vi "Error - Process.vi"(8 "error in (no error)":errorcluster, 11 "View Model":T1) -> (0 "error out":errorcluster)   [LabVIEW 2017]
doc: "Template for creating process"
uses:
  View Model/Controls/View Model.ctl
  Controls/Error Model.ctl
  Controls/Error EventData.ctl
  Controls/Error Type.ctl
  Elevator Controller/Controls/Elevator Model.ctl
  Elevator Controller/Controls/Elevator Overhead.ctl
  Elevator Controller/Controls/Elevator States.ctl
  Elevator Controller/Controls/Elevator Location.ctl
  Elevator Controller/Controls/Elevator Command Event.ctl
  Elevator Controller/Controls/Elevator Commands.ctl
  Configuration/Controls/Configuration Model.ctl
  Configuration/Controls/Configuration Data.ctl
  View Model/Controls/Shared Model.ctl
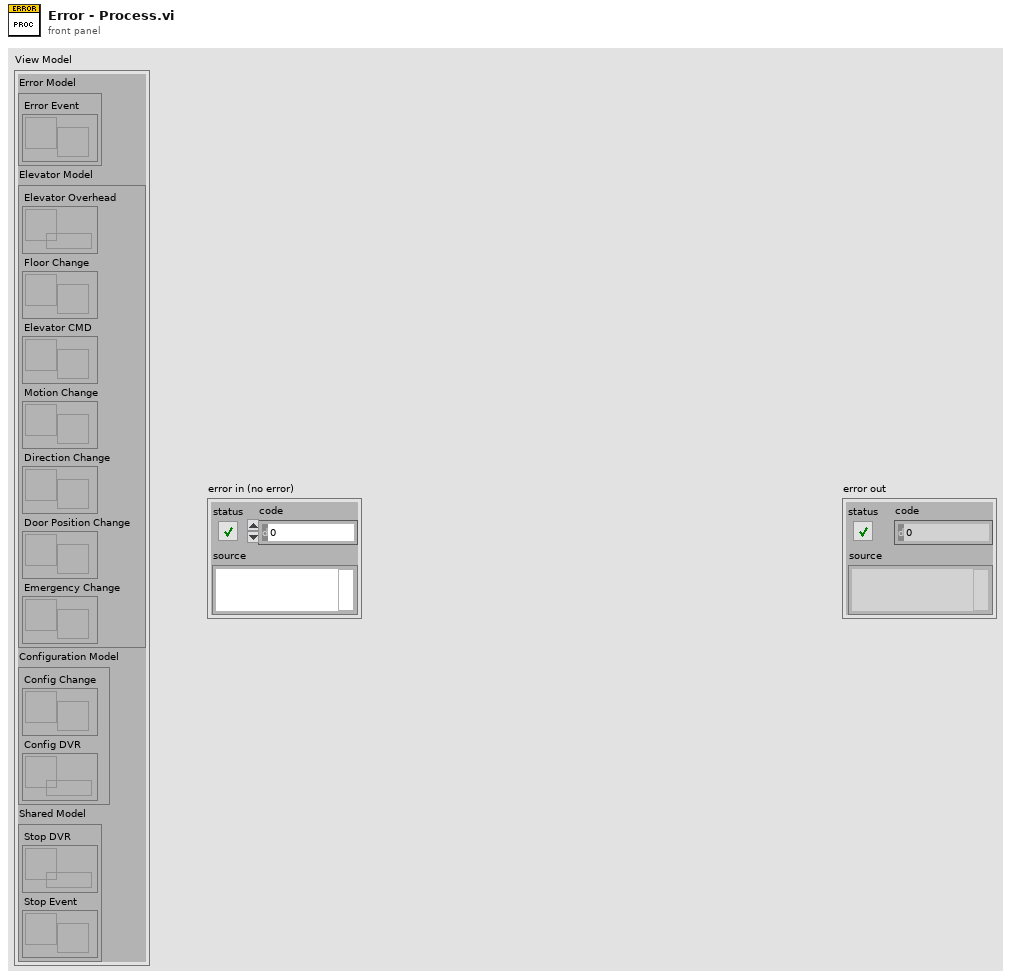
[diagram p1: front panel]
types:
  T1 = typedef "View Model.ctl" = cluster{"Error Model":T2, "Elevator Model":T3, "Configuration Model":T4, "Shared Model":T5}
  T2 = typedef "Error Model.ctl" = cluster{"Error Event":refnum<user-event>}
  T3 = typedef "Elevator Model.ctl" = cluster{"Elevator Overhead":refnum<data-value>, "Floor Change":refnum<user-event>, "Elevator CMD":refnum<user-event>, "Motion Change":refnum<user-event>, "Direction Change":refnum<user-event>, "Door Position Change":refnum<user-event>, "Emergency Change":refnum<user-event>}
  T4 = typedef "Configuration Model.ctl" = cluster{"Config Change":refnum<user-event>, "Config DVR":refnum<data-value>}
  T5 = typedef "Shared Model.ctl" = cluster{"Stop DVR":refnum<data-value>, "Stop Event":refnum<user-event>}
  T6 = typedef "Error Type.ctl" = enum16{"Console Error", "Sensor Interface IO Error", "Process Step Error"}
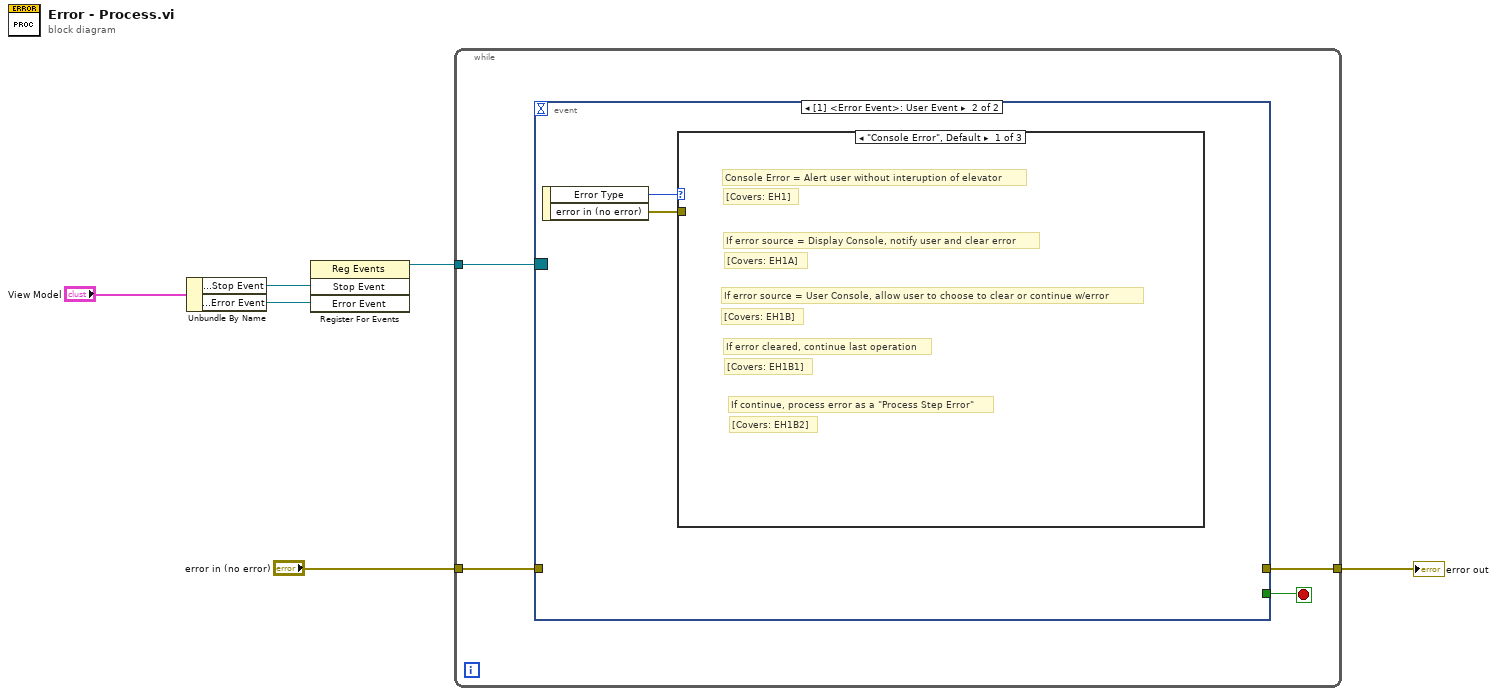
[diagram p0: block diagram]
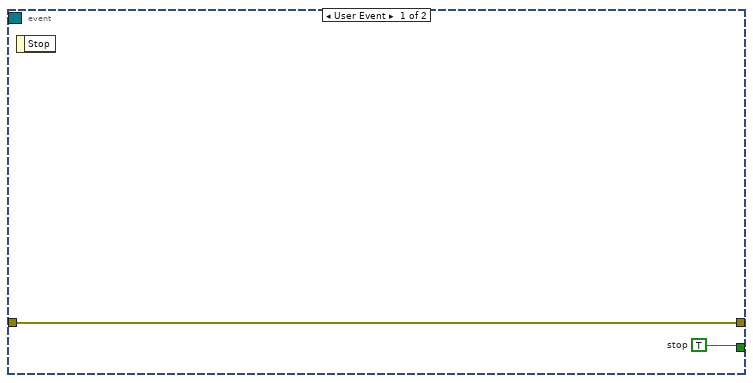
[diagram p2: hidden frame]
diagram:
  n1 = Unbundle By Name("View Model") -> ("Shared Model.Stop Event"=w5:refnum<user-event>, "Error Model.Error Event"=w4:refnum<user-event>)
  n2 = register-events(w5, w4) -> (reference out=w3:refnum<event-registration>)  [unwired: 2 in, 1 out]
  n3 = while {
    tunnel: w3 -> [w10]
    tunnel: "error in (no error)" -> [w9]
    tunnel: [w8] -> w1
    stop <- w7 stop-if-true
    n4 = event shown="[1] <Error Event>: User Event" {
      selector: w10 -> [_ _]
      dyn-events: _ -> [_ _]
      timeout: _ -> [_ _]
      tunnel: w9 -> [w12 _]
      tunnel: [w12 _] -> w8
      tunnel: [w11 _] -> w7
      event User Event {
        w11 = TRUE  # stop
        n5 = event-data() -> ()  [unwired: 1 in, 1 out]
      }
      event User Event {
        n6 = event-data() -> ("Error Type"=w14:T6, "error in (no error)"=w13:errorcluster)  [unwired: 1 in]
        n7 = case shown="\"Console Error\", Default" w14 {
          tunnel: w13 -> [_ _ _]
          frame "Console Error", Default {
            # "[Covers: EH1B2]"
            # "If continue, process error as a \"Process Step Error\""
            # "[Covers: EH1B1]"
            # "If error cleared, continue last operation"
            # "[Covers: EH1B]"
            # "If error source = User Console, allow user to choose to clear or continue w/error"
            # "[Covers: EH1A]"
            # "If error source = Display Console, notify user and clear error"
            # "[Covers: EH1]"
            # "Console Error = Alert user without interuption of elevator"
          }
          frame "Sensor Interface IO Error" {
            # "[Covers: EH2]"
            # "Execute termination process"
          }
          frame "Process Step Error" {
            # "[Covers: EH3]"
            # "Execute termination process"
          }
        }
      }
    }
  }
  "error out" <- w1
